vi "Toggle Output.vi"(8 "error in":errorcluster, 11 "6700C in":refnum<class "6700C.lvclass">) -> (0 "error out":errorcluster, 3 "6700C out":refnum<class "6700C.lvclass">)   [LabVIEW 2019, in "6700C.lvlib" / "6700C.lvclass"]
uses:
  Library/6700C.lvclass
  C:/Users/Public/Documents/Development/builds/Instruments/PowerSupply.lvlibp/Library/PowerSupply.lvclass
  Library/6700C.lvclass/6700C.ctl
  Accessors/Read Local Resource.vi
  Accessors/Write Local Resource.vi
  builds/Instruments/PowerSupply.lvlibp/Accessors/Read Active Channel.vi
  <instrlib>/Agilent N6700 Series/Agilent N6700 Series.lvlib
  builds/Engine/Engine.lvlibp/Project/Engine.lvclass
  C:/Users/Public/Documents/Development/builds/Engine/Engine.lvlibp/Project/Engine.lvclass
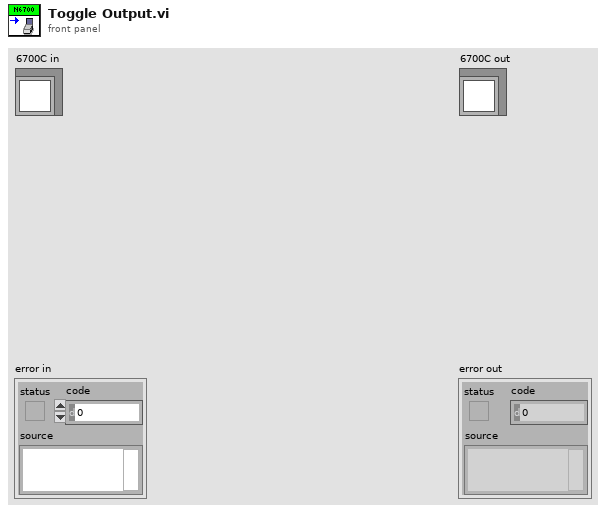
[diagram p1: front panel]
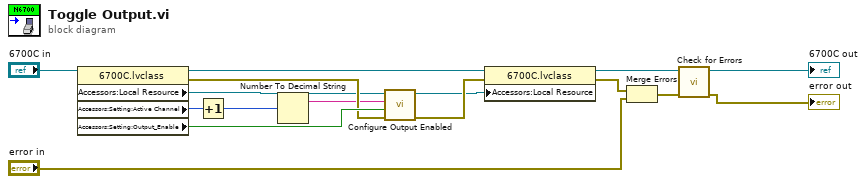
[diagram p0: block diagram]
diagram:
  n1 = property class="6700C.lvclass"(reference="6700C in") -> (reference out=w12:refnum<class "6700C.lvclass">, error out=w11:errorcluster, "Accessors:Local Resource"=w10:refnum<visa-resource-name>, "Accessors:Setting:Active Channel"=w15:u32, "Accessors:Setting:Output_Enable"=w16:bool)  [unwired: 1 in]
  n2 = Increment(x=w15) -> (x+1=w3:u32)
  n3 = Number To Decimal String(number=w3) -> (decimal integer string=w8:string)  [unwired: 1 in]
  n4 = call <instrlib>:"Configure Output Enabled.vi"("error in (no error)"=w11, "Enable Output (False)"=w16, "Channel Name (1)"=w8, "VISA resource name"=w10) -> ("error out"=w14:errorcluster, "VISA resource name out"=w13:refnum<visa-resource-name>)  [unwired: 6 in]
  n5 = property class="6700C.lvclass"(reference=w12, error in=w14, "Accessors:Local Resource"=w13) -> (reference out=w7:refnum<class "6700C.lvclass">, error out=w6:errorcluster)
  n6 = Merge Errors(w6, "error in") -> (w2:errorcluster)
  n7 = call "Check for Errors.vi"("error in"=w2, "Engine in"=w7) -> ("error out"=→"error out":errorcluster, "Engine out"=→"6700C out":refnum<class "6700C.lvclass">)  [unwired: 8 in]
